vi "Create (Pointer).vi"(8 "error in":errorcluster, 11 "pointer":i64) -> (0 "error out":errorcluster, 3 "Value out":refnum<class "Value.lvclass">)   [LabVIEW 2020, in "Value.lvlib" / "Value.lvclass"]
uses:
  Value.lvclass
  Value.lvclass/Value.ctl
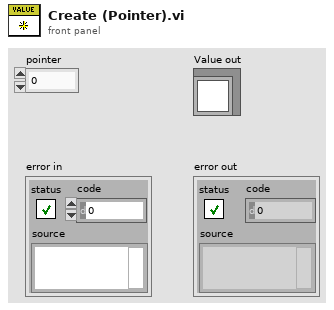
[diagram p1: front panel]
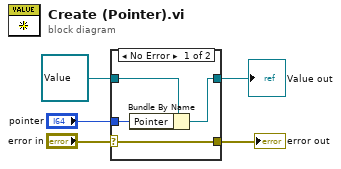
[diagram p0: block diagram]
diagram:
  n1 = case shown="No Error" "error in" {
    selector: "error in" -> [w7 w11]
    tunnel: [w7 w11] -> w5
    tunnel: refnum<class "Value.lvclass"> refnum ("Value in") -> [w9 w10]
    tunnel: [w8 w10] -> w2
    tunnel: "pointer" -> [w6 _]
    frame No Error {
      n2 = Bundle By Name(cluster=w9, "Pointer"=w6) -> (w8:refnum<class "Value.lvclass">)
    }
    frame Error {
    }
  }
  "error out" <- w5
  "Value out" <- w2
